vi "split_weights.vi"(11 "Output Layer Weights":T1(array[cluster])) -> (1 "Array 3":dbl[](array[numeric]), 2 "Array 2":dbl[](array[numeric]), 3 "Array":dbl[](array[numeric]))   [LabVIEW 2014]
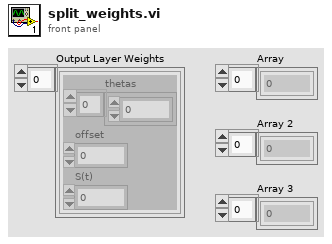
[diagram p1: front panel]
types:
  T1 = cluster{"thetas":dbl[], "offset":dbl, "S(t)":dbl}[]
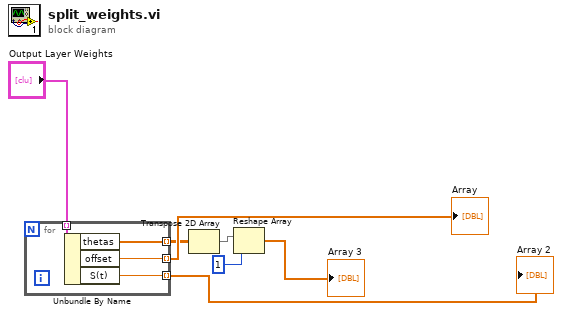
[diagram p0: block diagram]
diagram:
  n1 = for {
    tunnel: "Output Layer Weights" -> [w11] mode=indexing
    tunnel: [w10] -> w1 mode=indexing
    tunnel: [w9] -> w7 mode=indexing
    tunnel: [w8] -> w6 mode=indexing
    n2 = Unbundle By Name(w11) -> ("thetas"=w10:dbl[], "offset"=w9:dbl, "S(t)"=w8:dbl)
  }
  "Array" <- w7
  "Array 2" <- w6
  n3 = Transpose 2D Array(2D array=w1) -> (transposed array=w2:dbl[][])
  n4 = Reshape Array(w2, 1 ("dimension size")) -> (→"Array 3":dbl[])
